vi "Read States.vi"(8 "error in (no error)":errorcluster, 11 "DefendAreaTactic in":refnum<class "DefendAreaTactic.lvclass">) -> (0 "error out":errorcluster, 2 "States":T1, 3 "DefendAreaTactic out":refnum<class "DefendAreaTactic.lvclass">)   [LabVIEW 2024, in "DefendAreaTactic.lvclass"]
uses:
  DefendAreaTactic.lvclass
  DefendAreaTacticStates.ctl
  DefendAreaTactic.lvclass/DefendAreaTactic.ctl
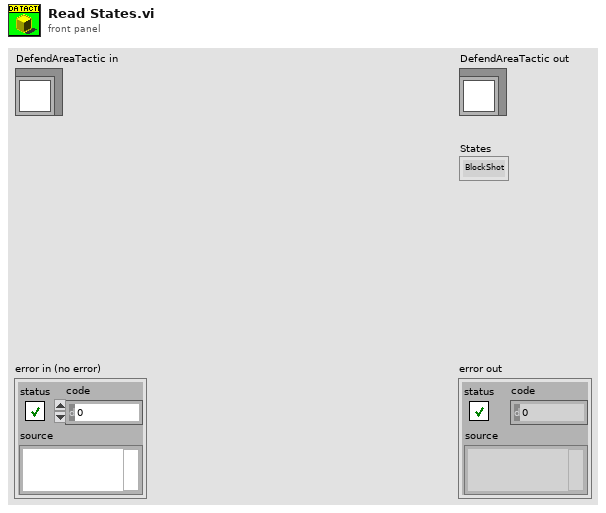
[diagram p1: front panel]
types:
  T1 = typedef "DefendAreaTactic.lvclass/DefendAreaTacticStates.ctl" = enum16{"BlockShot", "BlockPossibleShot", "CoverOneTouchShot", "BallInKeeperArea", "Exit"}
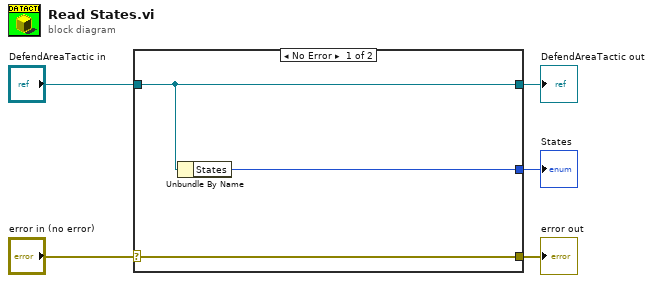
[diagram p0: block diagram]
diagram:
  n1 = case shown="No Error" "error in (no error)" {
    selector: "error in (no error)" -> [w8 w9]
    tunnel: [w8 w9] -> w4
    tunnel: [w7 w10] -> w2
    tunnel: "DefendAreaTactic in" -> [w7 w10]
    tunnel: [w6 _] -> w1
    frame No Error {
      n2 = Unbundle By Name(w7) -> ("States"=w6:T1)
    }
    frame Error {
    }
  }
  "error out" <- w4
  "DefendAreaTactic out" <- w2
  "States" <- w1
